vi "GetLimits.vi"(8 "error in (no error)":errorcluster, 11 "Stage_MadCityLab in":refnum<class "Stage_MadCityLab.lvclass">) -> (0 "error out":errorcluster, 1 "Lower Limit":dbl, 2 "Upper Limit":dbl, 3 "Stage_MadCityLab out":refnum<class "Stage_MadCityLab.lvclass">)   [LabVIEW 2020, in "Stage_MadCityLab.lvlib" / "Stage_MadCityLab.lvclass"]
uses:
  Stage_MadCityLab.lvclass
  HAL Layer/Stage/Stage/Stage.lvclass
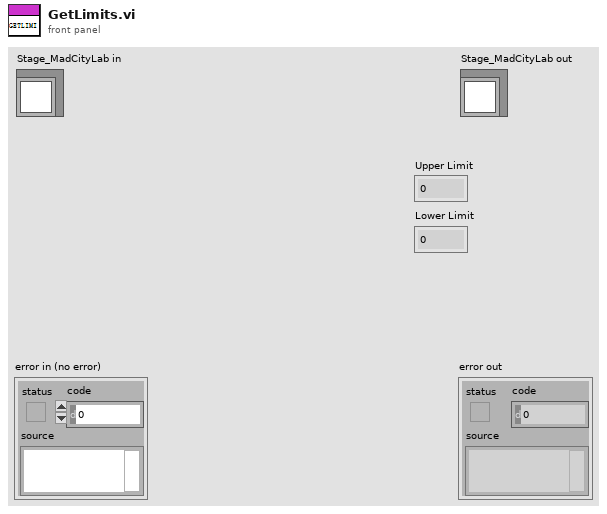
[diagram p1: front panel]
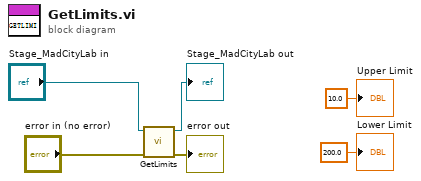
[diagram p0: block diagram]
diagram:
  n1 = call-parent "GetLimits.vi"("error in (no error)"="error in (no error)", "Stage in"="Stage_MadCityLab in") -> ("error out"=→"error out":errorcluster, "Stage out"=→"Stage_MadCityLab out":refnum<class "Stage_MadCityLab.lvclass">)  [unwired: 6 in, 2 out]
  "Upper Limit" <- 10.0 ("Upper Limit")
  "Lower Limit" <- 200.0 ("Lower Limit")
